vi "Demo_DataBase handling.vi"() -> ()   [LabVIEW 2017]
uses:
  <vilib>/addons/database/Connection.llb/DB Tools Open Connec (Path).vi
  <vilib>/addons/database/NI_Database_API.lvlib
panel:
  out "Data":string[][](array[string])
  in  "Read Database":bool
  in  "stop":bool
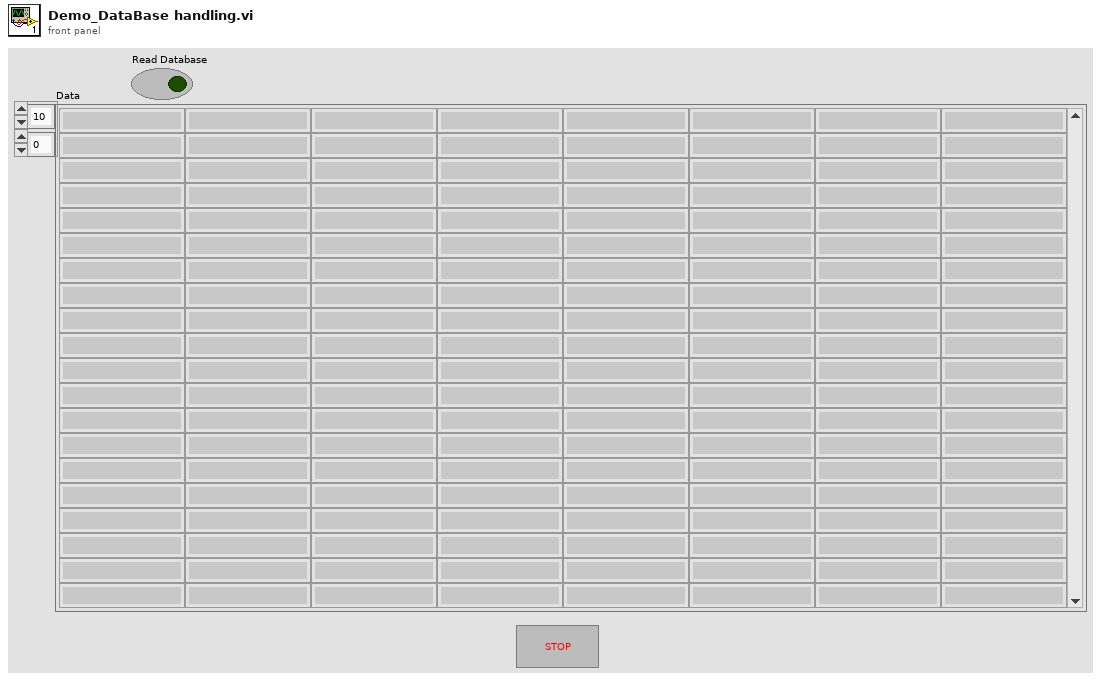
[diagram p1: front panel]
types:
  T1 = typedef "NI_Database_API.lvlib/Conn ObjectReference.ctl" = refnum<k1>
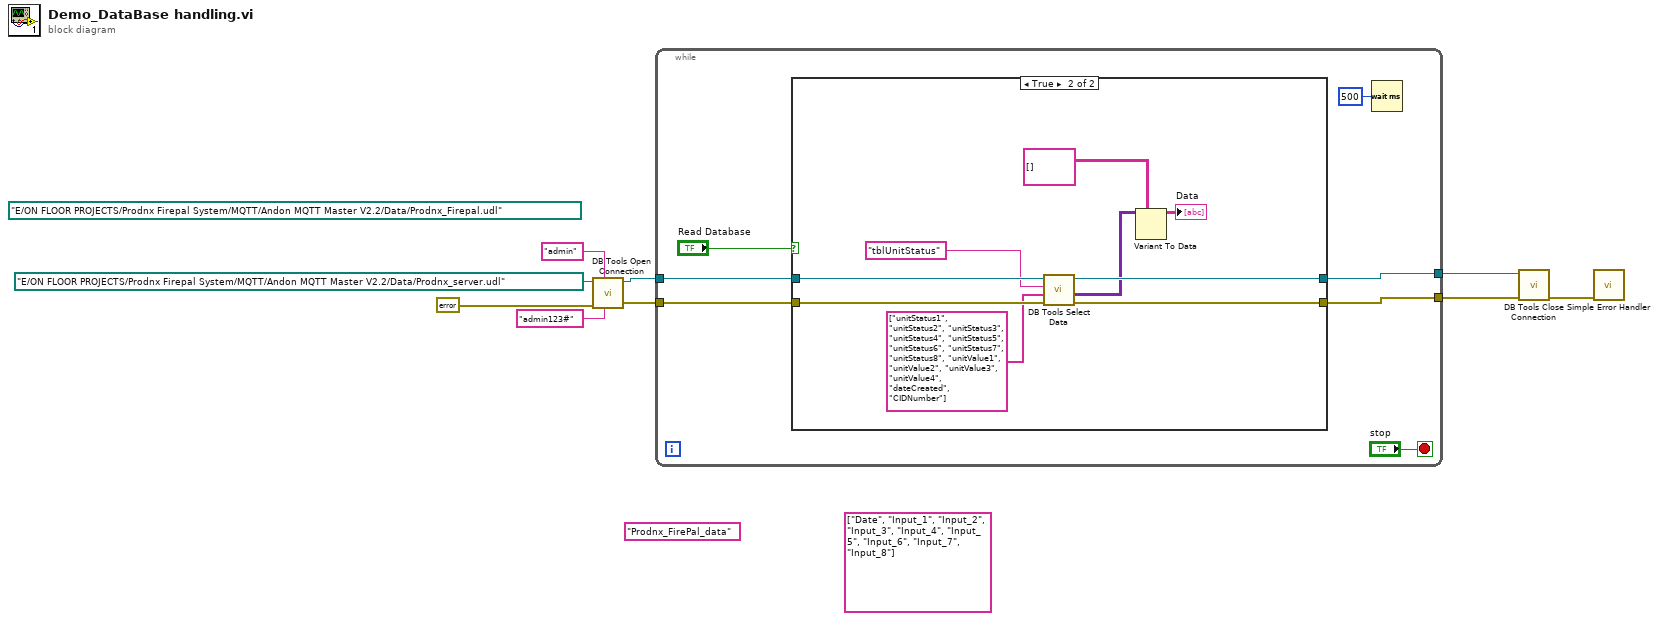
[diagram p0: block diagram]
diagram:
  (unwired) string[] ["Date", "Input_1", "Input_2", "Input_3", "Input_4", "Input_5", "Input_6", "Input_7", "Input_8"] ("columns")
  (unwired) "Prodnx_FirePal_data" ("table")
  (unwired) path "E:/ON FLOOR PROJECTS/Prodnx Firepal System/MQTT/Andon MQTT Master V2.2/Data/Prodnx_Firepal.udl" ("connection information")
  n1 = call-poly <vilib>:"DB Tools Open Connection.vi"("password"="admin123#", "userID"="admin", "error in (no error)"=errorcluster {"status"=FALSE, "code"=0, "source"=""}, "connection information"=path "E:/ON FLOOR PROJECTS/Prodnx Firepal System/MQTT/Andon MQTT Master V2.2/Data/Prodnx_server.udl") -> ("error out"=w7:errorcluster, "connection reference"=w8:T1)  [unwired: 4 in]
  n2 = while {
    tunnel: w8 -> [w14]
    tunnel: w7 -> [w13]
    tunnel: [w12] -> w6
    tunnel: [w11] -> w5
    stop <- "stop" stop-if-true
    n3 = case shown="True" "Read Database" {
      tunnel: w14 -> [w18 w27]
      tunnel: w13 -> [w17 w26]
      tunnel: [w18 w24] -> w12
      tunnel: [w17 w25] -> w11
      frame False {
      }
      frame True {
        n4 = call <vilib>:"DB Tools Select Data.vi"("error in (no error)"=w26, "columns"=string[] ["unitStatus1", "unitStatus2", "unitStatus3", "unitStatus4", "unitStatus5", "unitStatus6", "unitStatus7", "unitStatus8", "unitValue1", "unitValue2", "unitValue3", "unitValue4", "dateCreated", "CIDNumber"], "table"="tblUnitStatus", "connection reference"=w27) -> ("error out"=w25:errorcluster, "data"=w23:variant[][], "connection reference out"=w24:T1)  [unwired: 2 in]
        n5 = Variant To Data(type=string[][] [], Variant=w23) -> (data=→"Data":string[][])  [unwired: 1 in, 1 out]
      }
    }
    n6 = Wait (ms)(milliseconds to wait=u32 500) -> ()  [unwired: 1 out]
  }
  n7 = call <vilib>:"DB Tools Close Connection.vi"("error in (no error)"=w5, "connection reference"=w6) -> ("error out"=w4:errorcluster)  [unwired: 5 in]
  n8 = call <vilib>:"Simple Error Handler.vi"("error in (no error)"=w4) -> ()  [unwired: 4 in, 5 out]
